vi "Actor Core.vi"(8 "error in":errorcluster, 11 "RDS State Tracker in":refnum<class "RDS State Tracker.lvclass">) -> (0 "error out":errorcluster, 3 "Actor out":refnum<class "Actor.lvclass">)   [LabVIEW 2015, in "RDS State Tracker.lvlib" / "RDS State Tracker.lvclass"]
doc: "(<B>Filename</B>: Actor Framework.lvlib:Actor.lvclass:Actor Core.vi)\n\nReceives messages to the actor, reacts to them, and initiates any error handling that may shut the actor down.\n\nDescendant classes may override this VI to append parallel tasks for the actor to complete while it handles messages. Overrides use the Call Parent Method node."
uses:
  RDS State Tracker.lvclass
  <vilib>/ActorFramework/Actor/Actor.lvclass
  RDS State Tracker.lvclass/RDS State Tracker.ctl
  <vilib>/ActorFramework/Actor/Actor.lvclass/Actor.ctl
  <vilib>/ActorFramework/Message Enqueuer/Message Enqueuer.lvclass/Message Enqueuer.ctl
  <vilib>/ActorFramework/Message Enqueuer/Init from Existing Queue.vi
  <vilib>/ActorFramework/Message Enqueuer/Message Enqueuer.lvclass
  Actors/RDS Parent Actor/RDS Parent Actor/RDS Parent Actor.lvclass
  RDS State Tracker Messages/State Tracker Send Sample Msg/State Tracker Send Sample Msg.lvclass
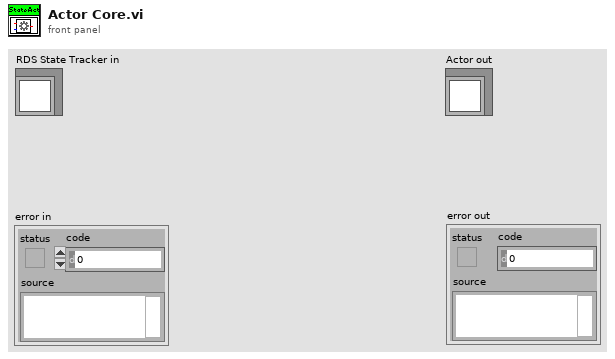
[diagram p1: front panel]
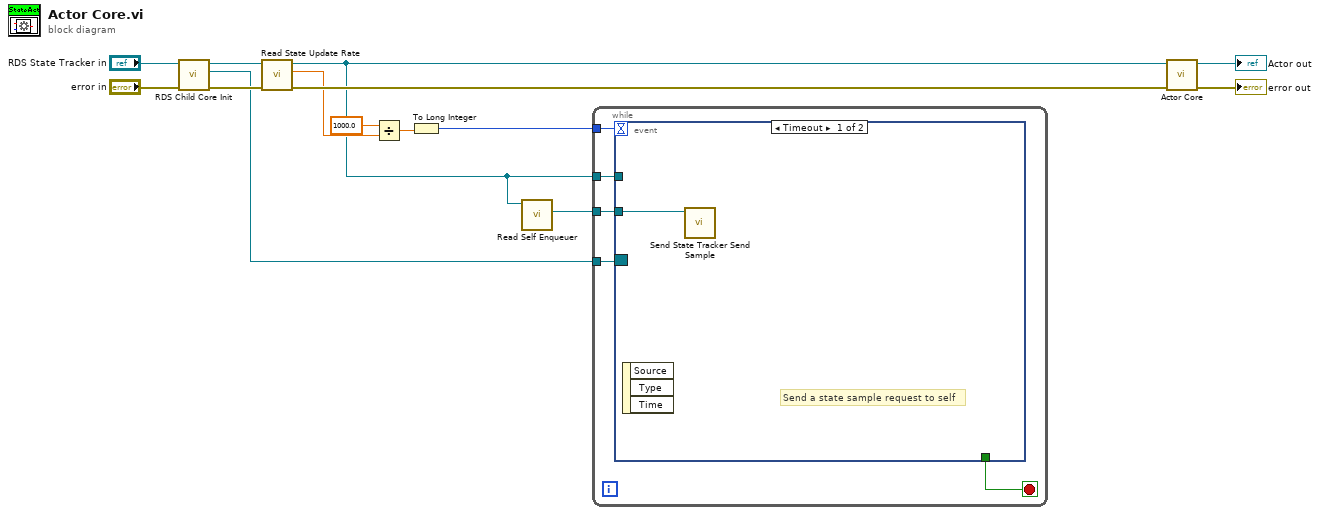
[diagram p0: block diagram]
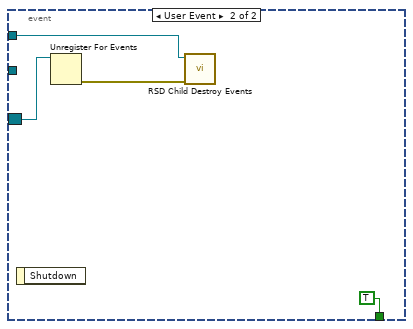
[diagram p2: hidden frame]
diagram:
  n1 = call "RDS Child Core Init.vi"("error in (no error)"="error in", "RDS Parent Actor in"="RDS State Tracker in") -> ("error out"=w9:errorcluster, "Event Registration Refnum"=w3:refnum<event-registration>, "RDS Parent Actor out"=w10:refnum<class "RDS State Tracker.lvclass">)  [unwired: 6 in, 1 out]
  n2 = call "Read State Update Rate.vi"("error in (no error)"=w9, "RDS State Tracker in"=w10) -> ("error out"=w8:errorcluster, "State Update Rate"=w6:dbl, "RDS State Tracker out"=w2:refnum<class "RDS State Tracker.lvclass">)  [unwired: 7 in]
  n3 = Divide(x=1000.0, y=w6) -> (x/y=w5:dbl)
  n4 = To Long Integer(number=w5) -> (32bit integer=w4:i32)
  n5 = call <vilib>:"Read Self Enqueuer.vi"("Actor"=w2) -> ("Self Enqueuer"=w1:refnum<class "Message Enqueuer.lvclass">)  [unwired: 10 in]
  n6 = while {
    tunnel: w3 -> [w18]
    tunnel: w2 -> [w19]
    tunnel: w4 -> [w16]
    tunnel: w1 -> [w15]
    stop <- w17 stop-if-true
    n7 = event shown="[0] Timeout" {
      selector: w18 -> [_ w22]
      dyn-events: _ -> [_ _]
      timeout: w16 -> [_ _]
      tunnel: w19 -> [_ w21]
      tunnel: [_ TRUE] -> w17
      tunnel: w15 -> [w20 _]
      event Timeout {
        # "Send a state sample request to self"
        n8 = event-data() -> ()  [unwired: 1 in, 3 out]
        n9 = call "Send State Tracker Send Sample.vi"("Message Enqueuer in"=w20) -> ()  [unwired: 9 in, 2 out]
      }
      event User Event {
        n10 = event-data() -> ()  [unwired: 1 in, 1 out]
        n11 = Unregister For Events(event registration refnum=w22) -> (error out=w23:errorcluster)  [unwired: 1 in]
        n12 = call "RSD Child Destroy Events.vi"("error in (no error)"=w23, "RDS Parent Actor in"=w21) -> ()  [unwired: 8 in, 2 out]
      }
    }
  }
  n13 = call-parent "Actor Core.vi"("error in"=w8, "Actor in"=w2) -> ("error out"=→"error out":errorcluster, "Actor out"=→"Actor out":refnum<class "Actor.lvclass">)  [unwired: 8 in]
